vi "getSettingsManager.vi"(8 "error in (no error)":errorcluster, 11 "CameraController.lvclass in":refnum<class "CameraController.lvclass">) -> (0 "error out":errorcluster, 2 "Tools.lvlib:Settings.lvlib:SettingsManager.lvclass":refnum<class "SettingsManager.lvclass">, 3 "CameraController.lvclass out":refnum<class "CameraController.lvclass">)   [LabVIEW 2009, in "Hardware.lvlib" / "Channels.lvlib" / "CameraController.lvclass"]
uses:
  CameraController.lvclass
  Tools/SettingsManager/SettingsManager.lvclass
  CameraController.lvclass/CameraController.ctl
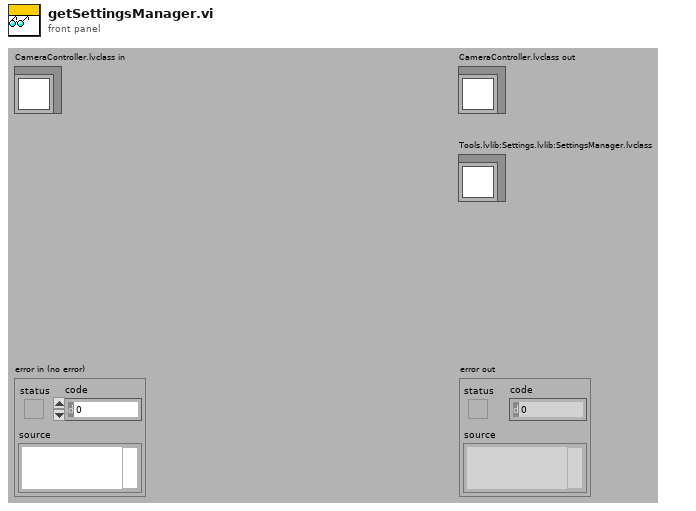
[diagram p1: front panel]
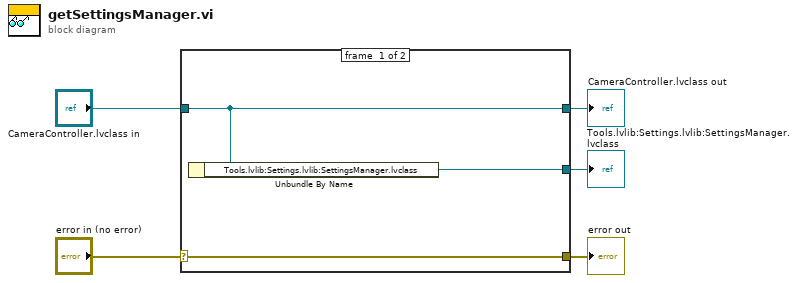
[diagram p0: block diagram]
diagram:
  n1 = case shown="No Error" "error in (no error)" {
    selector: "error in (no error)" -> [w8 w9]
    tunnel: [w8 w9] -> w4
    tunnel: [w7 w10] -> w2
    tunnel: "CameraController.lvclass in" -> [w7 w10]
    tunnel: [w6 _] -> w1
    frame #0 {
      n2 = Unbundle By Name(w7) -> ("Tools.lvlib:Settings.lvlib:SettingsManager.lvclass"=w6:refnum<class "SettingsManager.lvclass">)
    }
    frame #1 {
    }
  }
  "error out" <- w4
  "CameraController.lvclass out" <- w2
  "Tools.lvlib:Settings.lvlib:SettingsManager.lvclass" <- w1
